vi "SetAttributeViReal64.vi"(7 "AttributeValue":dbl, 8 "error in (no error)":errorcluster {"code" format="%.0x"}, 9 "AttributeID":u32(ring)=1150557 items=["ANALOGDEMODULATOR_CHANNEL_BANDWIDTH"=1150557, "ANALOGDEMODULATOR_TIME"=1150559, "ATTENUATION"=1250002, "DISPLAY_FREQUENCY_LINE               "=1150812, "DISPLAY_LINE"=1150191, "DISPLAY_NORMALIZED_REFERENCE"=1150184, "DISPLAY_REFERENCE_OFFSET"=1150186, "DISPLAY_REFERENCE"=1150185, "DISPLAY_Y_SCALE"=1150187, "EXTERNAL_MIXER_AVERAGE_CONVERSION_LOSS"=1250901, "EXTERNAL_MIXER_BIAS_LIMIT"=1250904, "EXTERNAL_MIXER_BIAS"=1250902, "EXTERNAL_TRIGGER_LEVEL"=1250401, "FREQUENCY_CENTER_STEP_INCREMENT"=1150541, "FREQUENCY_CENTER"=1150540, "FREQUENCY_OFFSET"=1250008, "FREQUENCY_SPAN_TO_RESOLUTION_BANDWIDTH_RATIO"=1150552, "FREQUENCY_SPAN"=1150542, "FREQUENCY_START"=1250006, "FREQUENCY_STOP"=1250007, "FREQUENCY_TRACE_ZOOM_CENTRE "=1150854, "FREQUENCY_TRACE_ZOOM_SPAN"=1150855, "FREQUENCY_ZONE_SPAN_CENTRE"=1150853, "FREQUENCY_ZONE_SPAN_SPAN"=1150868, "INPUT_IMPEDANCE"=1250009, "INPUT_RF_CENTER_FREQUENCY"=1150744, "INPUT_RF_CORRECTIONS_BASE_STATION_GAIN"=1150673, "INPUT_RF_CORRECTIONS_EXTERNAL_GAIN"=1150570, "INPUT_RF_CORRECTIONS_MOBILE_STATION_GAIN"=1150740, "INPUT_RF_MAX_MIXER_LEVEL"=1150572, "INPUT_RF_PEAK_TO_AVERAGE"=1150873, "INPUT_RF_RANGE"=1150872, "LEVEL_MIXER_OFFSET"=1150874], 10 "RepCapIdentifier":string, 11 "instrument handle":refnum<k15>) -> (0 "error out":errorcluster {"code" format="%.0x"}, 3 "instrument handle out":refnum<k15>)   [LabVIEW 2009, in "Keysight XSAn.lvlib"]
doc: "Sets a Real64 attribute from the instrument driver.\nThe following Attributes are supported:\n\nANALOGDEMODULATOR_CHANNEL_BANDWIDTH\nANALOGDEMODULATOR_TIME\nATTENUATION\nDISPLAY_FREQUENCY_LINE \nDISPLAY_LINE\nDISPLAY_NORMALIZED_REFERENCE\nDISPLAY_REFERENCE_OFFSET\nDISPLAY_REFERENCE\nDISPLAY_Y_SCALE\nEXTERNAL_MIXER_AVERAGE_CONVERSION_LOSS\nEXTERNAL_MIXER_BIAS_LIMIT\nEXTERNAL_MIXER_BIAS\nEXTERNAL_TRIGGER_LEVEL\nFREQUENCY_CENTER_STEP_INCREMENT\nFREQUENCY_CENTER\nFREQUENCY_OFFSET\nFREQUENCY_SPAN_TO_RESOLUTION_BANDWIDTH_RATIO\nFREQUENCY_SPAN\nFREQUENCY_START\nFREQUENCY_STOP\nFREQUENCY_TRACE_ZOOM_CENTRE \nFREQUENCY_TRACE_ZOOM_SPAN \nFREQUENCY_ZONE_SPAN_CENTRE \nFREQUENCY_ZONE_SPAN_SPAN \nINPUT_IMPEDANCE\nINPUT_RF_CENTER_FREQUENCY\nINPUT_RF_CORRECTIONS_BASE_STATION_GAIN\nINPUT_RF_CORRECTIONS_EXTERNAL_GAIN\nINPUT_RF_CORRECTIONS_MOBILE_STATION_GAIN\nINPUT_RF_MAX_MIXER_LEVEL\nINPUT_RF_PEAK_TO_AVERAGE \nINPUT_RF_RANGE \nLEVEL_MIXER_OFFSET"
uses:
  <instrlib>/Keysight XSAn/Keysight XSAn.lvlib
  AgXSAn.dll
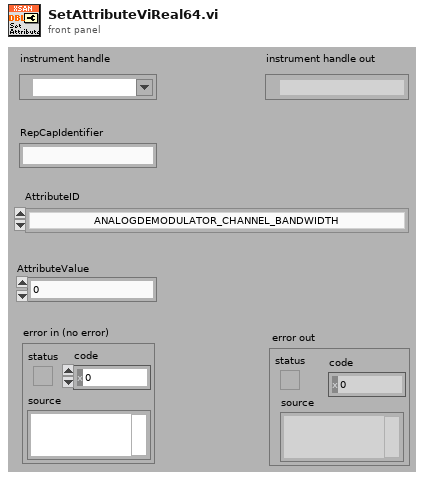
[diagram p1: front panel]
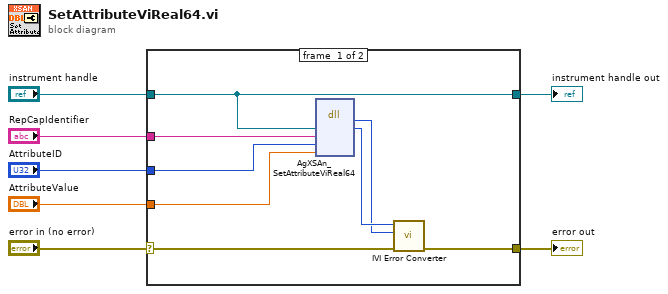
[diagram p0: block diagram]
diagram:
  n1 = case shown="No Error" "error in (no error)" {
    selector: "error in (no error)" -> [w13 w17]
    tunnel: [w12 w17] -> w7
    tunnel: "instrument handle" -> [w8 w16]
    tunnel: "RepCapIdentifier" -> [w11 _]
    tunnel: "AttributeID" -> [w10 _]
    tunnel: "AttributeValue" -> [w9 _]
    tunnel: [w8 w16] -> w1
    frame #0 {
      n2 = dll-call lib="AgXSAn**.dll" fn="AgXSAn_SetAttributeViReal64"("Vi"=w8, "RepCapIdentifier"=w11, "AttributeID"=w10, "AttributeValue"=w9) -> ("return type"=w14:i32, "Vi"=w15:u32)  [unwired: 6 in, 2 out]
      n3 = call <instrlib>:"IVI Error Converter.vi"("error in (no error)"=w13, "IVI error code (0)"=w14, "instrument handle"=w15) -> ("error out"=w12:errorcluster)  [unwired: 7 in, 1 out]
    }
    frame #1 {
    }
  }
  "error out" <- w7
  "instrument handle out" <- w1
